vi "Get Action Name.vi"(8 "error in (no error)":errorcluster, 11 "Action in":refnum<class "Action.lvclass">) -> (0 "error out":errorcluster, 2 "Action Name":string, 3 "Action out":refnum<class "Action.lvclass">)   [LabVIEW 2020, in "neg-pkg.lvlib" / "Action.lvclass"]
uses:
  Action.lvclass
  <vilib>/regexp/Match Regular Expression.xnode
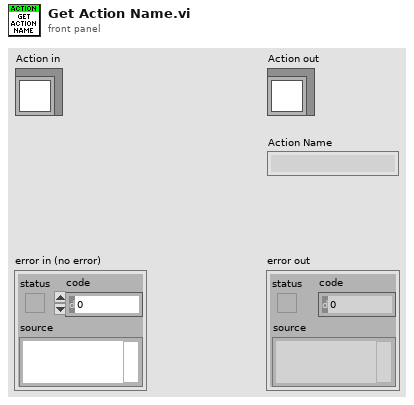
[diagram p1: front panel]
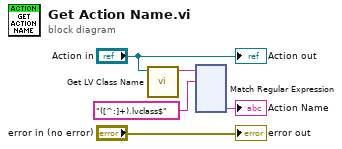
[diagram p0: block diagram]
diagram:
  n1 = call <vilib>:"Get LV Class Name.vi"("object"="Action in") -> ("class name"=w4:string)  [unwired: 9 in, 1 out]
  n2 = xnode "Match Regular Expression"("input string"=w4, "regular expression"="([^:]+).lvclass$") -> ("submatch 1"=→"Action Name":string)  [unwired: 4 in, 5 out]
  "error out" <- "error in (no error)"
  "Action out" <- "Action in"
